vi "create points in direction.vi"(9 "angle":dbl, 11 "distance":u32) -> (1 "x values":dbl[](array[numeric]), 3 "out-of-range point (y)":dbl)   [LabVIEW 2009]
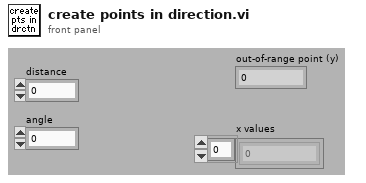
[diagram p1: front panel]
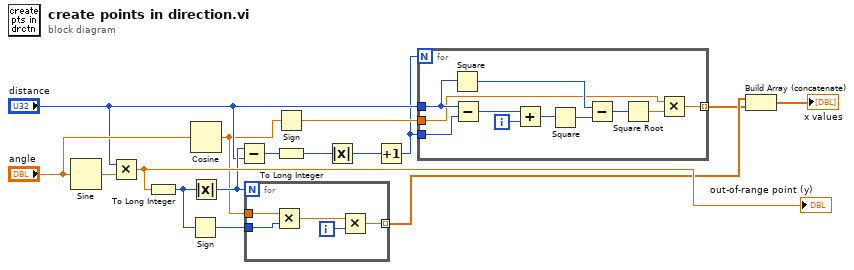
[diagram p0: block diagram]
diagram:
  n1 = Sine(x="angle") -> (sin(x)=w16:dbl)
  n2 = Multiply(x="distance", y=w16) -> (x*y=w15:dbl)
  "out-of-range point (y)" <- w15
  n3 = To Long Integer(number=w15) -> (32bit integer=w14:i32)
  n4 = Sign(1:w14) -> (0:w5:i32)
  n5 = Cosine(x="angle") -> (cos(x)=w4:dbl)
  n6 = Absolute Value(x=w14) -> (abs(x)=w12:i32)
  n7 = Subtract(x=w12, y="distance") -> (x-y=w9:u32)
  n8 = for {
    N: w12 -> [_]
    tunnel: w5 -> [w19]
    tunnel: w4 -> [w20]
    tunnel: [w17] -> w11 mode=indexing
    i -> [w21]
    n9 = Multiply(x=w20, y=w19) -> (x*y=w18:dbl)
    n10 = Multiply(x=w18, y=w21) -> (x*y=w17:dbl)
  }
  n11 = Sign(1:w4) -> (0:w3:dbl)
  n12 = To Long Integer(number=w9) -> (32bit integer=w8:i32)
  n13 = Absolute Value(x=w8) -> (abs(x)=w7:i32)
  n14 = Increment(x=w7) -> (x+1=w1:i32)
  n15 = for {
    N: w1 -> [_]
    tunnel: "distance" -> [w32]
    tunnel: [w27] -> w2 mode=indexing
    tunnel: w3 -> [w26]
    tunnel: w1 -> [w22]
    i -> [w24]
    n16 = Square(x=w32) -> (x^2=w31:u32)
    n17 = Subtract(x=w32, y=w22) -> (x-y=w25:u32)
    n18 = Add(x=w25, y=w24) -> (x+y=w23:u32)
    n19 = Square(x=w23) -> (x^2=w30:u32)
    n20 = Subtract(x=w31, y=w30) -> (x-y=w29:u32)
    n21 = Square Root(x=w29) -> (sqrt(x)=w28:dbl)
    n22 = Multiply(x=w26, y=w28) -> (x*y=w27:dbl)
  }
  n23 = Build Array (concatenate)(w11, w2) -> (→"x values":dbl[])
